vi "Init.vi"(7 "Connection State":refnum<notifier>, 8 "error in (no error)":errorcluster, 9 "Client List":refnum<notifier>, 10 "Msg Handlers":refnum<queue>, 11 "Send Queue":refnum<queue>) -> (0 "error out":errorcluster, 3 "TCPMessageService out":refnum<class "TCPMessageAPI.lvclass">)   [LabVIEW 2020, in "Vecto.lvlib" / "TCPMessageAPI.lvclass"]
uses:
  TCPMessageAPI.lvclass
  Send Message Data.ctl
  proto/TcpPayload/Data.ctl
  lv-promises/Promises/Promise/Promise.lvclass
  TCPMessageHandler/TCPMessageHandler.lvclass
  proto/TcpClientList/Data.ctl
  proto/TcpClientInfo/Data.ctl
  TCPMessageAPI.lvclass/TCPMessageAPI.ctl
  proto/TcpPayload/TcpPayload.lvlib
  Vecto.lvlib
  proto/TcpClientInfo/TcpClientInfo.lvlib
  proto/TcpClientList/TcpClientList.lvlib
  Connected Status.ctl
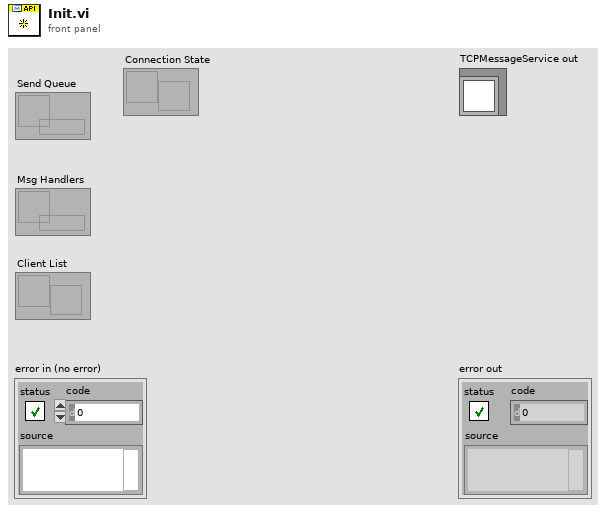
[diagram p1: front panel]
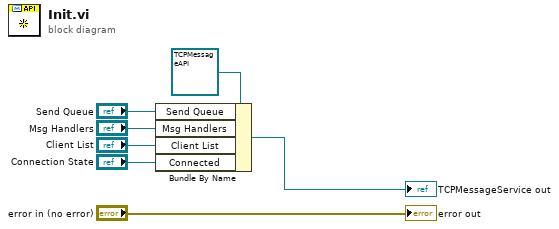
[diagram p0: block diagram]
diagram:
  n1 = Bundle By Name(cluster=refnum<class "TCPMessageAPI.lvclass"> refnum ("TCPMessageService in"), "Send Queue"="Send Queue", "Msg Handlers"="Msg Handlers", "Client List"="Client List", "Connected"="Connection State") -> (→"TCPMessageService out":refnum<class "TCPMessageAPI.lvclass">)
  "error out" <- "error in (no error)"
